vi "用户登录.vi"(8 "error in (no error)":errorcluster caption="错误输入（无错误）", 9 "Password":string caption="密   码:", 11 "UserName":string caption="用户名:") -> (0 "error out":errorcluster caption="错误输出", 1 "ErrorMessage":string, 2 "登录成功":bool)   [LabVIEW 2015]
uses:
  mes/ctl/SenduserRightVerify.ctl
  mes/ctl/ReceiveuserRightVerify.ctl
  Global.vi
panel:
  in  "Headers":string[][](array[string])=[["Content-Type", "text/xml;charset=UTF-8"], ["SOAPAction", "\"http://tempuri.org/IUserRightVerifyServiceImpl/UserRightVerify\""], ["Connection", "Keep-Alive"], ["User-Agent", "Apache-HttpClient/4.1.1 (java 1.5)"]]
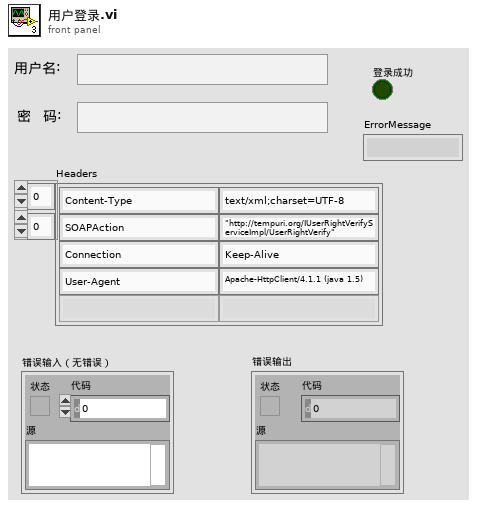
[diagram p1: front panel]
types:
  T1 = typedef "SenduserRightVerify.ctl" = cluster{"#attributes":cluster{"xmlns:soapenv":string, "xmlns:tem":string, "xmlns:cal":string}, "soapenv:Header":string, "soapenv:Body":cluster{"tem:UserRightVerify":cluster{"tem:model":cluster{"cal:equipNum":string, "cal:passWord":string, "cal:siteCode":string, "cal:userName":string}}}}
  T2 = cluster{"接口地址(URL)":string, "权限校验":string, "产品进站":string, "参数采集":string, "产品出站":string, "设备状态":string, "设备编号(equipNum)":string, "站点名称(siteCode)":string, "生产类型(productType)":string, "试验单号(testOrderNum)":string}
  T3 = typedef "ReceiveuserRightVerify.ctl" = cluster{"#attributes":cluster{"xmlns:s":string}, "s:Body":cluster{"UserRightVerifyResponse":cluster{"#attributes":cluster{"xmlns":string}, "UserRightVerifyResult":cluster{"#attributes":cluster{"xmlns:a":string, "xmlns:i":string}, "a:ErrorCode":string, "a:ErrorMessage":string, "a:Success":string}}}}
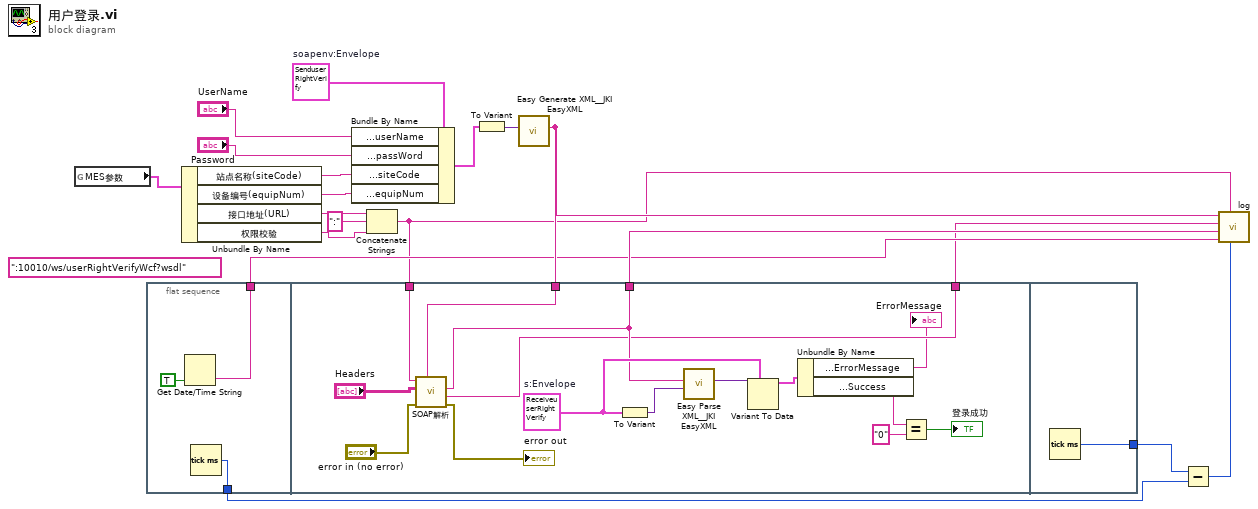
[diagram p0: block diagram]
diagram:
  w4 = T1 {"#attributes"={"xmlns:soapenv"="http://schemas.xmlsoap.org/soap/envelope/", "xmlns:tem"="http://tempuri.org/", "xmlns:cal"="http://schemas.datacontract.org/2004/07/CalbUserRightVerifyService"}, "soapenv:Header"="", "soapenv:Body"={"tem:UserRightVerify"={"tem:model"={"cal:equipNum"="", "cal:passWord"="", "cal:siteCode"="", "cal:userName"=""}}}}  # soapenv:Envelope
  (unwired) ":10010/ws/userRightVerifyWcf?wsdl"
  n1 = global read "Global.vi" "MES参数"() -> (w15:T2)
  n2 = flat-sequence {
    tunnel: [w22] -> w10
    tunnel: [w20] -> w7
    tunnel: w5 -> [w37]
    tunnel: w9 -> [w27]
    tunnel: [w26] -> w8
    tunnel: [w25] -> w3
    tunnel: [w38] -> w11
    frame #0 {
      n3 = Get Date/Time String(want seconds? (F)=TRUE ("需要秒？(F)")) -> (time string=w20:string)  [unwired: 2 in, 1 out]
      n4 = Tick Count (ms)() -> (millisecond timer value=w22:u32)
    }
    frame #1 {
      w29 = T3 {"#attributes"={"xmlns:s"="http://schemas.xmlsoap.org/soap/envelope/"}, "s:Body"={"UserRightVerifyResponse"={"#attributes"={"xmlns"="http://tempuri.org/"}, "UserRightVerifyResult"={"#attributes"={"xmlns:a"="http://schemas.datacontract.org/2004/07/EdgeUtility", "xmlns:i"="http://www.w3.org/2001/XMLSchema-instance"}, "a:ErrorCode"="", "a:ErrorMessage"="", "a:Success"=""}}}}  # s:Envelope
      n5 = call "SOAP解析.vi"("DATA"=w27, "错误输入（无错误）"="error in (no error)", "Headers"="Headers", "URL"=w37) -> ("错误输出"=→"error out":errorcluster, "headers"=w25:string, "body"=w26:string)  [unwired: 5 in]
      n6 = To Variant(anything=w29) -> (Variant=w36:variant)
      n7 = call <vilib>:"Easy Parse XML__JKI EasyXML.vi"("LabVIEW Data (Type)"=w36, "XML String"=w26) -> ("LabVIEW Data"=w35:variant)  [unwired: 8 in, 1 out]
      n8 = Variant To Data(type=w29, Variant=w35) -> (data=w34:T3)  [unwired: 1 in, 1 out]
      n9 = Unbundle By Name(w34) -> ("s:Body.UserRightVerifyResponse.UserRightVerifyResult.a:ErrorMessage"=→"ErrorMessage":string, "s:Body.UserRightVerifyResponse.UserRightVerifyResult.a:Success"=w33:string)
      n10 = Equal?(x=w33, y="0") -> (x = y?=→"登录成功":bool)
    }
    frame #2 {
      n11 = Tick Count (ms)() -> (millisecond timer value=w38:u32)
    }
  }
  n12 = Unbundle By Name(w15) -> ("站点名称(siteCode)"=w16:string, "设备编号(equipNum)"=w17:string, "接口地址(URL)"=w12:string, "权限校验"=w1:string)
  n13 = Bundle By Name(cluster=w4, "soapenv:Body.tem:UserRightVerify.tem:model.cal:userName"="UserName", "soapenv:Body.tem:UserRightVerify.tem:model.cal:passWord"="Password", "soapenv:Body.tem:UserRightVerify.tem:model.cal:siteCode"=w16, "soapenv:Body.tem:UserRightVerify.tem:model.cal:equipNum"=w17) -> (w19:T1)
  n14 = Concatenate Strings(w12, ":" ("字符串"), w1) -> (w5:string)
  n15 = To Variant(anything=w19) -> (Variant=w18:variant)
  n16 = call <vilib>:"Easy Generate XML__JKI EasyXML.vi"("LabVIEW Data"=w18) -> ("XML String"=w9:string)  [unwired: 9 in, 1 out]
  n17 = Subtract(x=w11, y=w10) -> (x-y=w6:u32)
  n18 = call "log.vi"("接口耗时"=w6, "URL"=w5, "StartTime"=w7, "响应报文"=w8, "header"=w3, "发送报文"=w9) -> ()  [unwired: 6 in]
